vi "Find API Tester Path.vi"(8 "error in":errorcluster, 11 "Event vi Ref":refnum<vi>) -> (0 "error out":errorcluster, 3 "API Tester Path":path)   [LabVIEW 2020, in "DQMH_API.lvlib"]
uses:
  DQMH_API.lvlib
  <vilib>/ErrorRing/Error Ring.xnode
  <vilib>/Utility/error.llb/Error Cluster From Error Code.vi
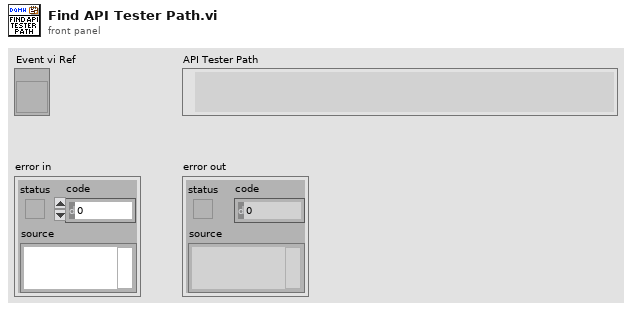
[diagram p1: front panel]
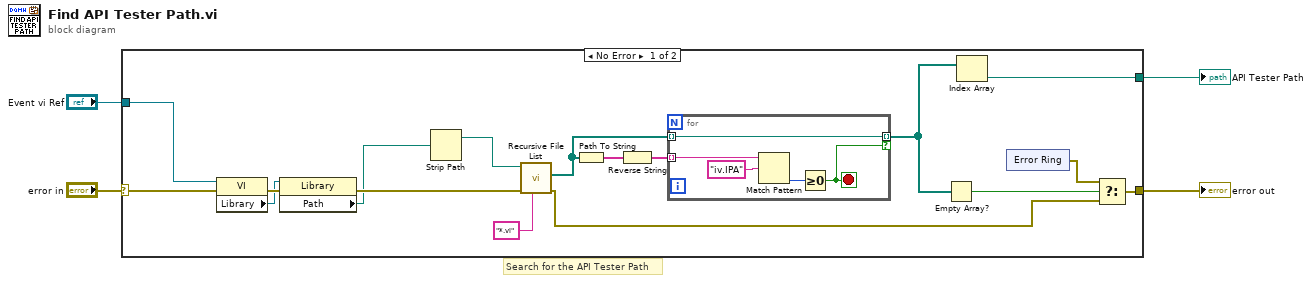
[diagram p0: block diagram]
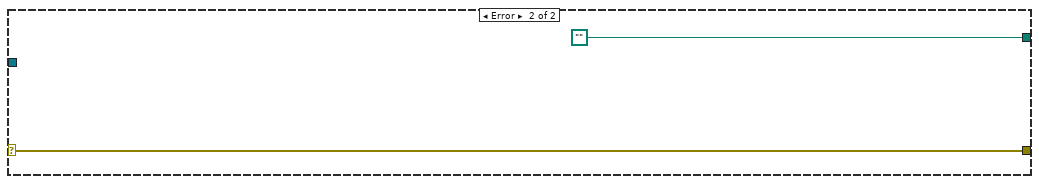
[diagram p2: hidden frame]
diagram:
  # "Search for the API Tester Path"
  n1 = case shown="No Error" "error in" {
    selector: "error in" -> [w17 w33]
    tunnel: [w11 path ""] -> w2
    tunnel: [w19 w33] -> w3
    tunnel: "Event vi Ref" -> [w5 _]
    frame No Error {
      n2 = property class="VI"(reference=w5, error in=w17) -> (error out=w18:errorcluster, "Library"=w7:refnum<vi>)  [unwired: 1 out]
      n3 = property class="Library"(reference=w7, error in=w18) -> (error out=w16:errorcluster, "Path"=w6:path)  [unwired: 1 out]
      n4 = Strip Path(path=w6) -> (stripped path=w8:path)  [unwired: 1 out]
      n5 = call <vilib>:"Recursive File List.vi"("pattern"="*.vi", "error in (no error)"=w16, "Folder Path"=w8) -> ("error out"=w20:errorcluster, "All Files in Dir"=w12:path[])  [unwired: 4 in, 3 out]
      n6 = Path To String(path=w12) -> (string=w14:string[])
      n7 = Reverse String(1:w14) -> (0:w13:string[])
      n8 = for {
        tunnel: w13 -> [w29] mode=indexing
        tunnel: w12 -> [w31] mode=indexing
        tunnel: [w31] -> w10 mode=indexing if=w27
        stop <- w27 stop-if-true
        n9 = Match Pattern(string=w29, regular expression="iv.IPA") -> (offset past match=w28:i32)  [unwired: 1 in, 3 out]
        n10 = Greater Or Equal To 0?(x=w28) -> (x >= 0?=w27:bool)
      }
      n11 = Empty Array?(array=w10) -> (empty?=w9:bool)
      n12 = Index Array(array=w10) -> (element=w11:path)  [unwired: 1 in]
      n13 = xnode "Error Ring"() -> ("error out"=w21:errorcluster)
      n14 = Select(t=w21, s=w9, f=w20) -> (s? t:f=w19:errorcluster)
    }
    frame Error {
    }
  }
  "API Tester Path" <- w2
  "error out" <- w3
